vi "array.vi"() -> ()   [LabVIEW 2013]
panel:
  out "indeksy min lok":i32[](array[numeric])
  in  "stop":bool
  in  "tab liczb R":dbl[](array[numeric])
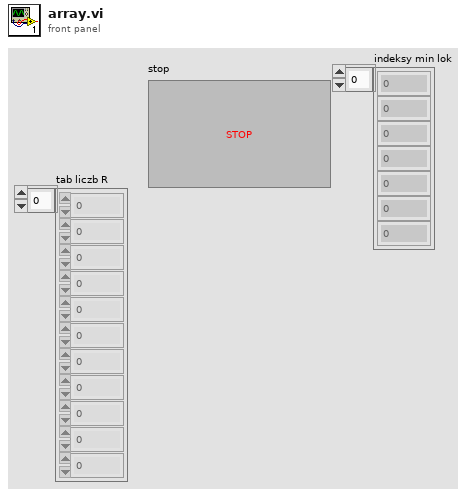
[diagram p1: front panel]
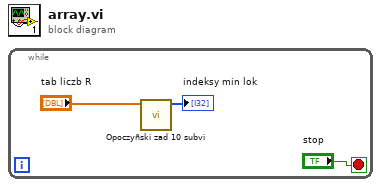
[diagram p0: block diagram]
diagram:
  n1 = while {
    stop <- "stop" stop-if-true
    n2 = call "Opoczyñski zad 10 subvi.vi"("tab liczb R"="tab liczb R") -> ("indeks"=→"indeksy min lok":i32[])  [unwired: 10 in]
  }
